vi "Get Voltage Resolution.vi"(8 "error in (no error)":errorcluster, 11 "channel":i8) -> (0 "error out":errorcluster, 3 "function return":dbl)   [LabVIEW 2023, in "vmmsolib.lvlib"]
doc: "DLL_API double WINAPI GetVoltageResolution(char channel);"
uses:
  vmmsolib.lvlib
  vmmso.dll
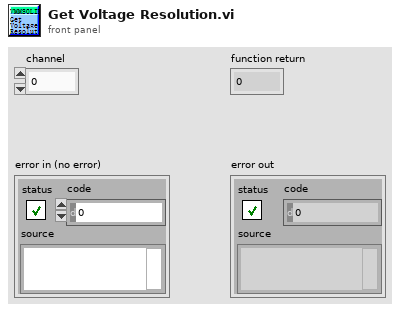
[diagram p1: front panel]
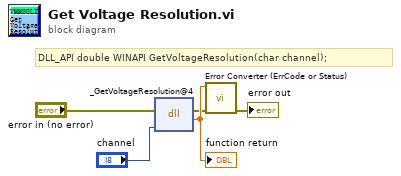
[diagram p0: block diagram]
diagram:
  # "DLL_API double WINAPI GetVoltageResolution(char channel);"
  n1 = dll-call lib="D:/VmMsoSDK/demo-Labview/2023/vmmsolib/vmmso.*" fn="_GetVoltageResolution@4"(error in="error in (no error)", "channel"="channel") -> (error out=w2:errorcluster, w5:dbl)  [unwired: 3 in, 1 out]
  "function return" <- w5
  n2 = call "Error Converter (ErrCode or Status).vi"("error in (no error)"=w2, "error code"=w5) -> ("error out"=→"error out":errorcluster)  [unwired: 9 in]
